vi "ZLIB Store File With CompressionLevels__ogtk.vi"(4 "password (none)":string, 5 "local extra data":string, 6 "-1: use default\ncompression":i32=-1, 7 "global extra data":string, 8 "error in (no error)":errorcluster, 9 "internal name (same as source name)":path, 10 "source path":path, 11 "zip Refnum":T2) -> (0 "error out":errorcluster, 3 "zip Refnum out":T2)   [LabVIEW 2013]
doc: "Adds a file to an archive in a zip session."
uses:
  <userlib>/_OpenG.lib/lvzip/lvzip.llb/ZLIB Zip Handle__ogtk.ctl
  <userlib>/_OpenG.lib/lvzip/lvzip.llb/ZLIB File Info__ogtk.ctl
panel:
  in  "file info":T1={"version"=0, "version needed"=0, "encrypted"=FALSE, "flag"=4294967295, "compression"=0, "dos date"=0, "crc"=0, "compressed size"=0, "uncompressed size"=0, "extra info"="", "file comment"="", "disk num start"=0, "internal fa"=0, "external fa"=0, "file timestamp"=0} {"file timestamp" format="%<%H:%M:%S\n%d/%m/%Y>T"; "external fa" format="%.0x"; "internal fa" format="%.0x"; "crc" format="%.0x"}
  # "Please visit http://www.OpenG.org to learn about the\nOpen Source LabVIEW software movement.\n\nNOTICE -- YOU MUST LEAVE THIS NOTICE IN PLACE.  PER THE TERMS OF THE LICENSE BELOW, YOU MAY SUBLICENSE THIS SOFTWARE \nIN ANY WAY THAT DOES NOT CONFLICT WITH THIS LICENSE.\n\n### BSD License (http://www.opensource.org/licenses/bsd-license.php) Begin ###\n \nCopyright (C) 2002-2004 Rolf Kalbermatter rolf.kalbermatter@citeng.com\nCopyright (C) 2002 Jim Kring jim@jimkring.com\n\nAll rights reserved.\n\nRedistribution and use in source and binary forms, with or without modification, are permitted provided that the following conditions are met:\n\n    * Redistributions of source code must retain the above copyright notice, this list of conditions and the following disclaimer.\n    * Redistributions in binary form must reproduce the above copyright notice, this list of conditions and the following disclaimer in the \n       documentation and/or other materials provided with the distribution.\n    * Neither the name of SciWare, James Kring, Inc., nor the names of its contributors may be used to endorse or promote products derived \n       from this software without specific prior written permission.\n\nTHIS SOFTWARE IS PROVIDED BY THE COPYRIGHT HOLDERS AND CONTRIBUTORS \"AS IS\" AND ANY EXPRESS OR IMPLIED WARRANTIES, \nINCLUDING, BUT NOT LIMITED TO, THE IMPLIED WARRANTIES OF MERCHANTABILITY AND FITNESS FOR A PARTICULAR PURPOSE ARE \nDISCLAIMED. IN NO EVENT SHALL THE COPYRIGHT OWNER OR CONTRIBUTORS BE LIABLE FOR ANY DIRECT, INDIRECT, INCIDENTAL,\n SPECIAL, EXEMPLARY, OR CONSEQUENTIAL DAMAGES (INCLUDING, BUT NOT LIMITED TO, PROCUREMENT OF SUBSTITUTE GOODS OR \nSERVICES; LOSS OF USE, DATA, OR PROFITS; OR BUSINESS INTERRUPTION) HOWEVER CAUSED AND ON ANY THEORY OF LIABILITY, \nWHETHER IN CONTRACT, STRICT LIABILITY, OR TORT (INCLUDING NEGLIGENCE OR OTHERWISE) ARISING IN ANY WAY OUT OF THE USE \nOF THIS SOFTWARE, EVEN IF ADVISED OF THE POSSIBILITY OF SUCH DAMAGE.\n\n### BSD License End ###"
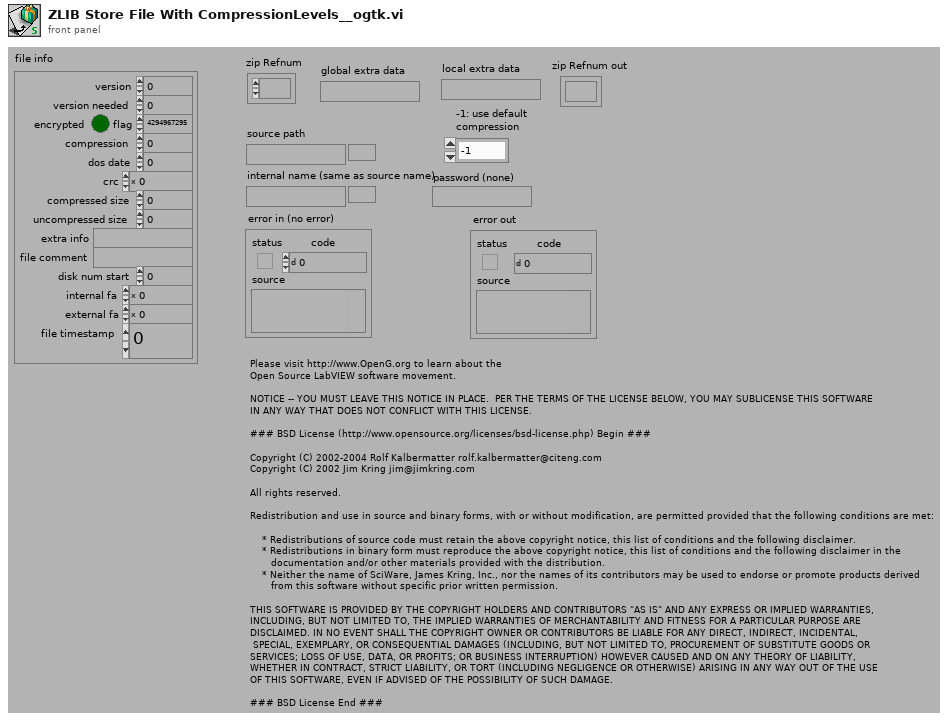
[diagram p1: front panel]
types:
  T1 = typedef "ZLIB File Info__ogtk.ctl" = cluster{"version":u32, "version needed":u32, "encrypted":bool, "flag":u32, "compression":i32, "dos date":u32, "crc":u32, "compressed size":u32, "uncompressed size":u32, "extra info":string, "file comment":string, "disk num start":u32, "internal fa":u32, "external fa":u32, "file timestamp":u32}
  T2 = typedef "ZLIB Zip Handle__ogtk.ctl" = refnum<k1>
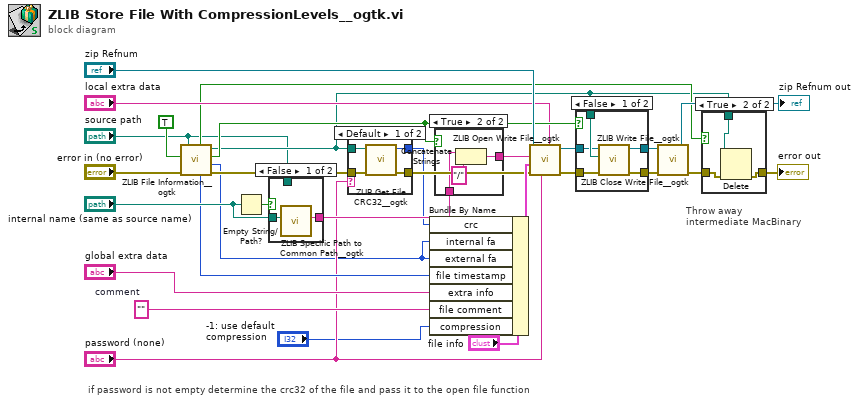
[diagram p0: block diagram]
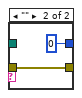
[diagram p3: hidden frame]
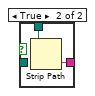
[diagram p5: hidden frame]
diagram:
  w14 = ""  # comment
  # "Throw away\nintermediate MacBinary"
  # "if password is not empty determine the crc32 of the file and pass it to the open file function"
  n1 = call <userlib>:"ZLIB File Information__ogtk.vi"("file path"="source path", "encode MacBinary (F)"=TRUE, "error in (no error)"="error in (no error)") -> ("created macbinary"=w4:bool, "file timestamp"=w13:u32, "file path out"=w2:path, "directory"=w19:bool, "file attributes"=w8:u32, "error out"=w9:errorcluster)  [unwired: 1 in]
  n2 = Empty String/Path?(string/path="internal name (same as source name)") -> (empty?=w23:bool)
  n3 = case shown="False" w23 {
    tunnel: "internal name (same as source name)" -> [w32 _]
    tunnel: [w31 w34] -> w21
    tunnel: "source path" -> [_ w33]
    frame False {
      n4 = call <userlib>:"ZLIB Specific Path to Common Path__ogtk.vi"("specific path"=w32) -> ("common path"=w31:string)  [unwired: 10 in]
    }
    frame True {
      n5 = Strip Path(path=w33) -> (name=w34:string)  [unwired: 1 out]
    }
  }
  n6 = case shown="Default" "password (none)" {
    tunnel: w9 -> [w38 w40]
    tunnel: [w37 w40] -> w11
    tunnel: [w36 u32 0 ("crc")] -> w10
    tunnel: w2 -> [w35 _]
    frame Default {
      n7 = call <userlib>:"ZLIB Get File CRC32__ogtk.vi"("error in (no error)"=w38, "file path"=w35) -> ("error out"=w37:errorcluster, "file crc32"=w36:u32)  [unwired: 4 in]
    }
    frame "" {
    }
  }
  n8 = Bundle By Name(cluster="file info", "crc"=w10, "internal fa"=w8, "external fa"=w8, "file timestamp"=w13, "extra info"="global extra data", "file comment"=w14, "compression"="-1: use default\ncompression") -> (w16:T1)
  n9 = case shown="True" w19 {
    tunnel: w21 -> [w41 w43]
    tunnel: [w41 w44] -> w20
    frame False {
    }
    frame True {
      n10 = Concatenate Strings(w43, "/" ("Format String")) -> (w44:string)
    }
  }
  n11 = call <userlib>:"ZLIB Open Write File__ogtk.vi"("local extra data"="local extra data", "password (none)"="password (none)", "error in (no error)"=w11, "file info"=w16, "filename"=w20, "zip Refnum"="zip Refnum") -> ("error out"=w27:errorcluster, "zip Refnum out"=w25:T2)  [unwired: 4 in]
  n12 = case shown="False" w19 {
    tunnel: [w49 w50] -> w29
    tunnel: w2 -> [w48 _]
    tunnel: w27 -> [w47 w50]
    tunnel: w25 -> [w46 w51]
    tunnel: [w45 w51] -> w24
    frame False {
      n13 = call <userlib>:"ZLIB Write File__ogtk.vi"("error in (no error)"=w47, "source path"=w48, "zip Refnum"=w46) -> ("error out"=w49:errorcluster, "zip Refnum out"=w45:T2)  [unwired: 4 in]
    }
    frame True {
    }
  }
  n14 = call <userlib>:"ZLIB Close Write File__ogtk.vi"("error in (no error)"=w29, "zip Refnum"=w24) -> ("error out"=w6:errorcluster, "zip Refnum out"=→"zip Refnum out":T2)  [unwired: 4 in]
  n15 = case shown="True" w4 {
    tunnel: w6 -> [w52 w55]
    tunnel: [w52 w54] -> w5
    tunnel: w2 -> [_ w53]
    frame False {
    }
    frame True {
      n16 = Delete(path (use dialog)=w53, error in=w55) -> (error out=w54:errorcluster)  [unwired: 3 in, 2 out]
    }
  }
  "error out" <- w5
